vi "Configure LAN Link.vi"(0 "VISA resource name":refnum<visa-resource-name>, 1 "Link Timeout (20 S)":dbl=20.0, 2 "Enable Nagle Algorithm (F: Disable)":bool, 5 "LXI Domain (0)":i32, 7 "Duplex Mode (1: Full-duplex)":i32(ring)=1 items=["Half-duplex ", "Full-duplex"], 9 "LAN Speed (1: 100 Mbps)":i32(ring)=1 items=["10 Mbps", "100 Mbps"], 11 "error in (no error)":errorcluster, 12 "Time Interval (20 S)":dbl=20.0) -> (4 "VISA resource name out":refnum<visa-resource-name>, 15 "error out":errorcluster)   [LabVIEW 2019, in "Keithley 2600 Series.lvlib"]
doc: "Configures the basic settings of the LAN link."
uses:
  Keithley 2600 Series.lvlib
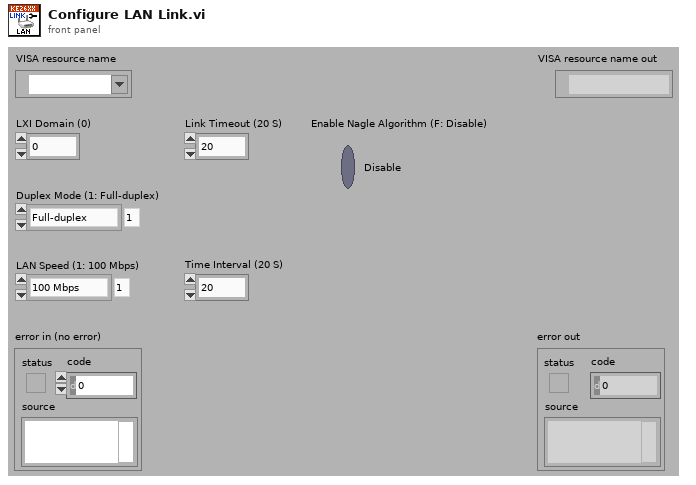
[diagram p1: front panel]
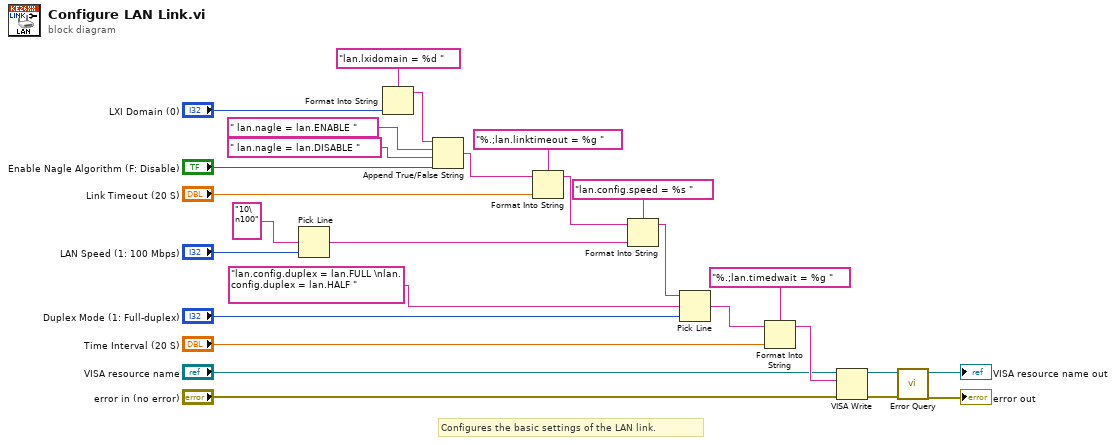
[diagram p0: block diagram]
diagram:
  # "Configures the basic settings of the LAN link."
  n1 = Pick Line(multi-line string="10\n100", line index="LAN Speed (1: 100 Mbps)") -> (output string=w1:string)  [unwired: 1 in]
  n2 = Format Into String(format string="lan.lxidomain = %d ", "LXI Domain (0)") -> (resulting string=w25:string)  [unwired: 2 in, 1 out]
  n3 = Append True/False String(1:"Enable Nagle Algorithm (F: Disable)", 2:" lan.nagle = lan.DISABLE ", 3:" lan.nagle = lan.ENABLE ", 4:w25) -> (0:w21:string)
  n4 = Format Into String(format string="%.;lan.linktimeout = %g ", initial string=w21, "Link Timeout (20 S)") -> (resulting string=w18:string)  [unwired: 1 in, 1 out]
  n5 = Format Into String(format string="lan.config.speed = %s ", initial string=w18, w1) -> (resulting string=w14:string)  [unwired: 1 in, 1 out]
  n6 = Pick Line(string ("")=w14, multi-line string="lan.config.duplex = lan.FULL \nlan.config.duplex = lan.HALF ", line index="Duplex Mode (1: Full-duplex)") -> (output string=w13:string)
  n7 = Format Into String(format string="%.;lan.timedwait = %g ", initial string=w13, "Time Interval (20 S)") -> (resulting string=w10:string)  [unwired: 1 in, 1 out]
  n8 = VISA Write(VISA resource name="VISA resource name", write buffer=w10, error in (no error)="error in (no error)") -> (VISA resource name out=w7:refnum<visa-resource-name>, error out=w6:errorcluster)  [unwired: 1 out]
  n9 = call "Error Query.vi"("error in (no error)"=w6, "VISA resource name"=w7) -> ("error out"=→"error out":errorcluster, "VISA resource name out"=→"VISA resource name out":refnum<visa-resource-name>)  [unwired: 6 in, 2 out]
